vi "test4.2-AsyncMessageWithReply_Queue.vi"(8 "error in (no error)":errorcluster, 11 "TestCase in":refnum<class "testcase-CSMGlobalLog.lvclass">) -> (0 "error out":errorcluster, 3 "TestCase out":refnum<class "testcase-CSMGlobalLog.lvclass">)   [LabVIEW 2017, in "testcase-CSMGlobalLog.lvclass"]
uses:
  testcase-CSMGlobalLog.lvclass
  testcase-CSMGlobalLog.lvclass/testcase-CSMGlobalLog.ctl
  c9cb4a92-c6b2-48ff-9945-b938079fd949.vi
  <vilib>/addons/_JKI Toolkits/VI Tester/TestCase.llb/TestCase.lvclass
  src/user.lib/_NEVSTOP/Communicable State Machine(CSM)/Communicable State Machine.lvlib
  src/user.lib/_NEVSTOP/Communicable State Machine(CSM)/Utility/Periodic String Filter Setting.ctl
  C:/Program Files (x86)/National Instruments/LabVIEW 2017/vi.lib/addons/_JKI Toolkits/VI Tester/TestCase.llb/TestCase.lvclass
panel:
  out "String cache total":string
  out "size(s)":i32
  out "error out 2":errorcluster
  out "LoopCount":i32
  out "String Cache each loop":string
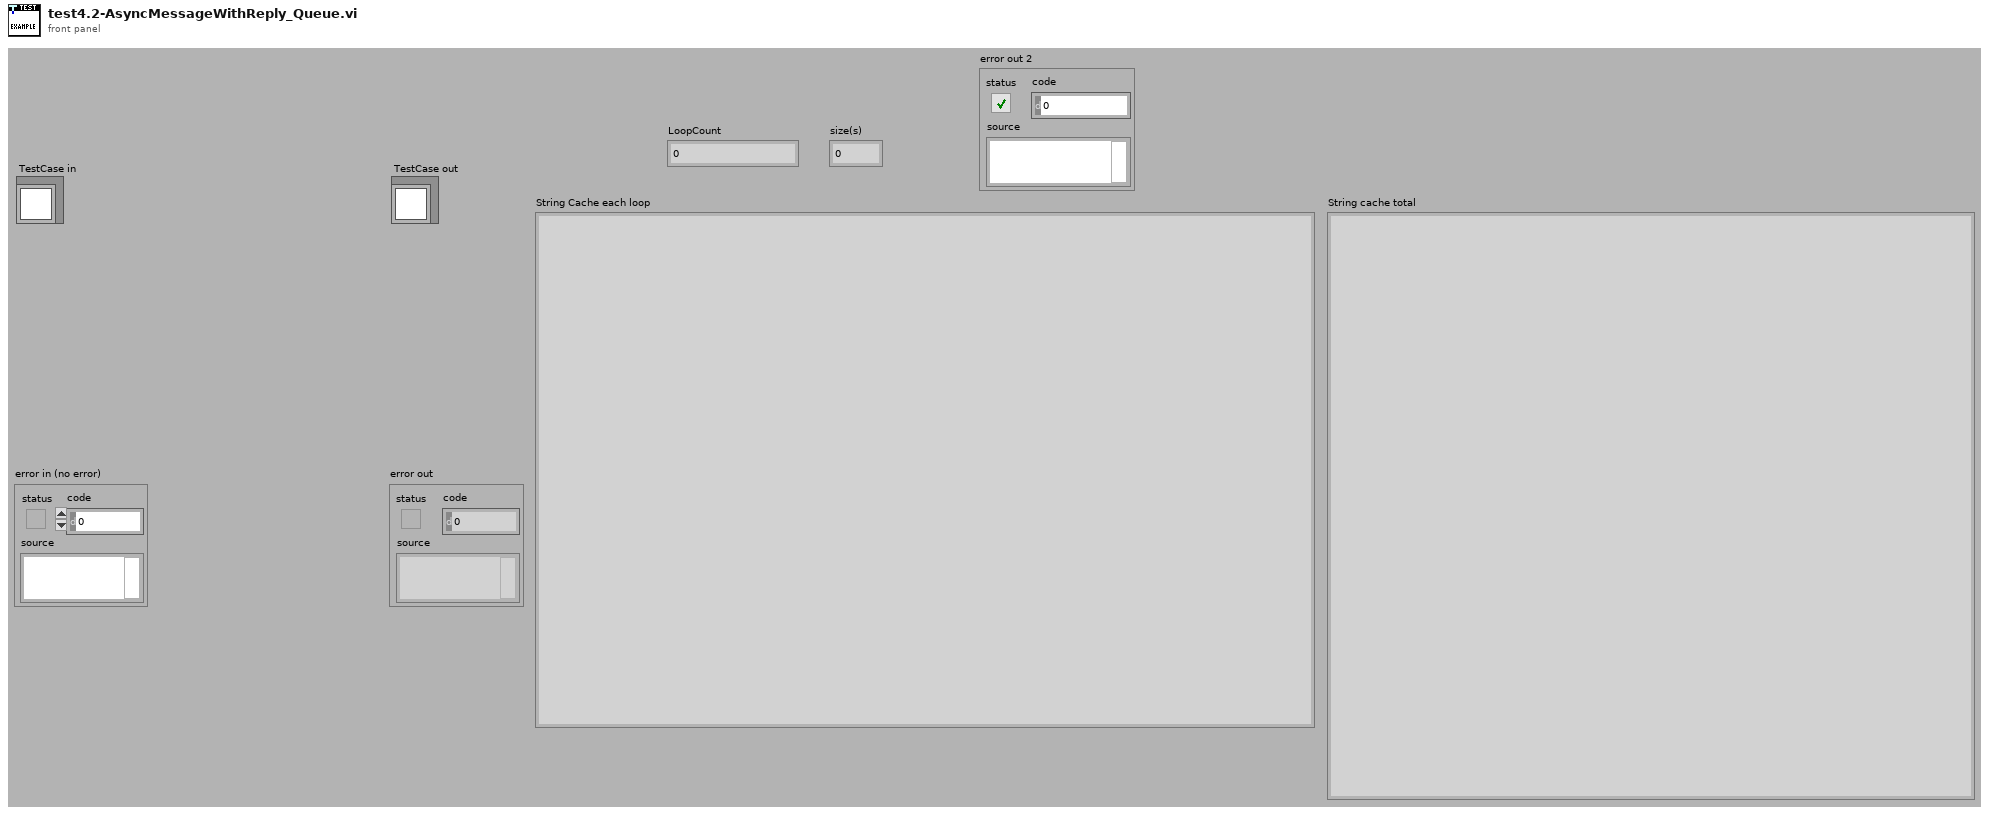
[diagram p1: front panel]
types:
  T1 = typedef "Communicable State Machine.lvlib/Periodic String Filter Setting.ctl" = cluster{"threashold(#/s)":dbl, "Check Peroid(s)":dbl}
  T2 = typedef "Communicable State Machine.lvlib/_CSM_GlobalLog_MSG.ctl" = cluster{"Name (\"\" to Use UUID)":string, "Current State":string, "Arguments":string, "Source Message":T3, "Source Module":string, "Complete(T)/Start(F)":bool, "LogType":T4, "Time Stamp":timestamp}
  T3 = typedef "Communicable State Machine.lvlib/_CSM_Response Source Message.ctl" = cluster{"‘State":string, "’Arguments":string, "’Error":errorcluster}
  T4 = typedef "Communicable State Machine.lvlib/_CSM_GlobalLog_MSG_TYPE.ctl" = enum16{"User Log", "State Change", "Status", "Interrupt", "Register", "Unregister", "Error Log", "Module Created", "Module Destroyed", "Async Message", "No-Rep Async Message", "Sync Message"}
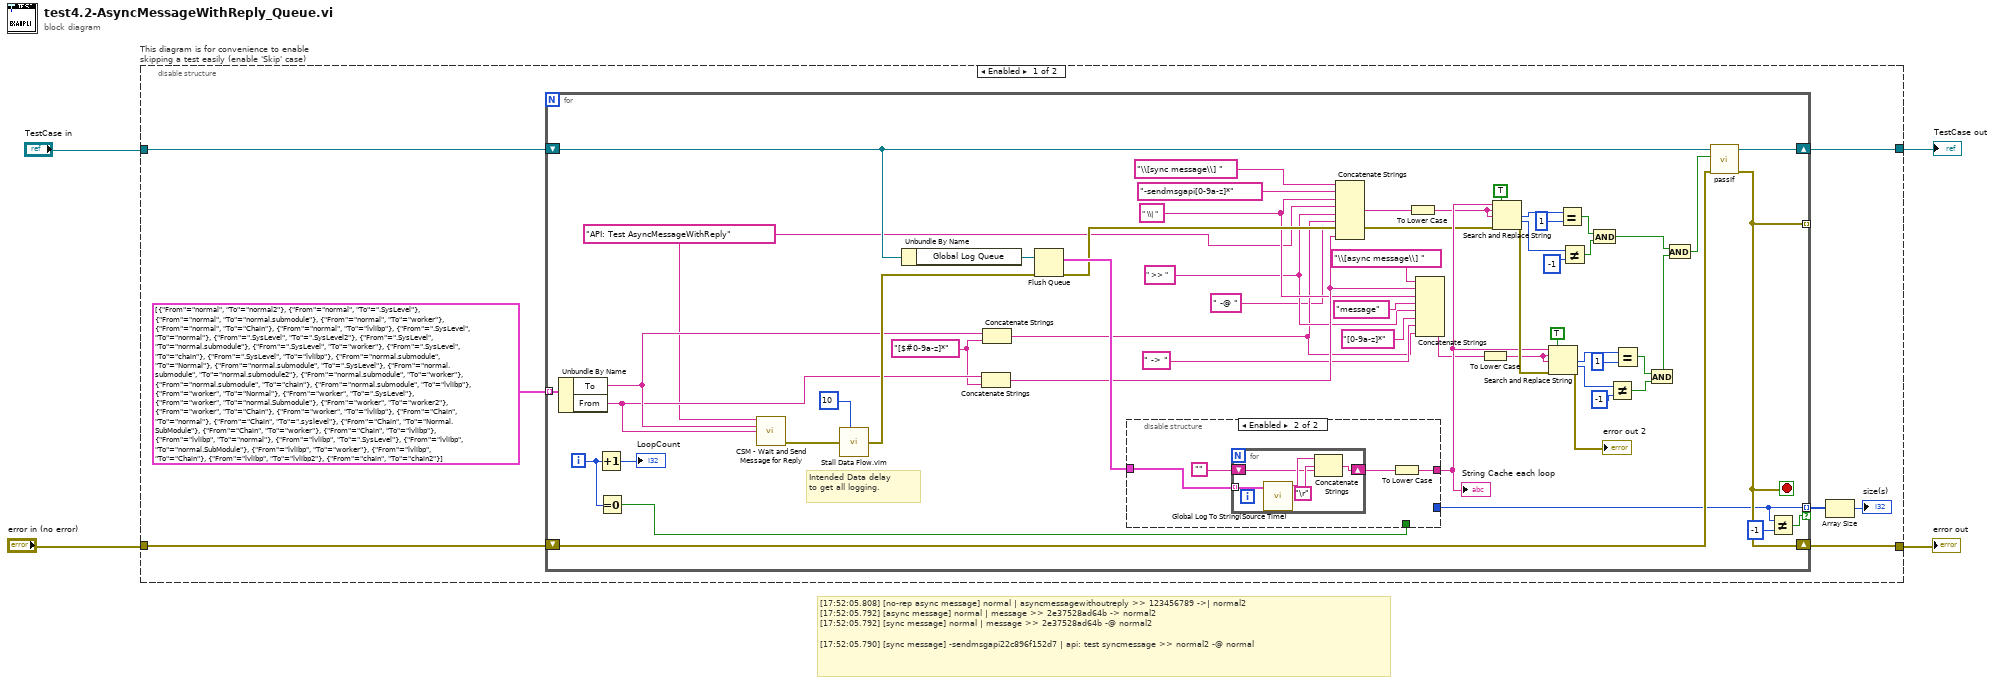
[diagram p0: block diagram]
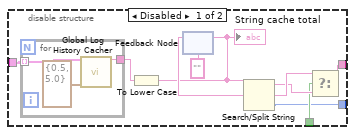
[diagram p2: hidden frame]
diagram:
  # "[17:52:05.808] [no-rep async message] normal | asyncmessagewithoutreply >> 123456789 ->| normal2\n[17:52:05.792] [async message] normal | message >> 2e37528ad64b -> normal2\n[17:52:05.792] [sync message] normal | message >> 2e37528ad64b -@ normal2\n\n[17:52:05.790] [sync message] -sendmsgapi22c896f152d7 | api: test syncmessage >> normal2 -@ normal"
  n1 = disable-structure "This diagram is for convenience to enable skipping a test easily (enable 'Skip' case)" shown="Enabled" {
    disable-tunnel: "TestCase in" -> [w8 w93]
    disable-tunnel: [w10 w91] -> w1
    disable-tunnel: [w11 w92] -> w3
    disable-tunnel: "error in (no error)" -> [w9 w90]
    frame Enabled {
      n2 = for {
        tunnel: cluster{"From":string, "To":string}[] [{"From"="normal", "To"="normal2"}, {"From"="normal", "To"=".SysLevel"}, {"From"="normal", "To"="normal.submodule"}, {"From"="normal", "To"="worker"}, {"From"="normal", "To"="Chain"}, {"From"="normal", "To"="lvlibp"}, {"From"=".SysLevel", "To"="normal"}, {"From"=".SysLevel", "To"=".SysLevel2"}, {"From"=".SysLevel", "To"="normal.submodule"}, {"From"=".SysLevel", "To"="worker"}, {"From"=".SysLevel", "To"="chain"}, {"From"=".SysLevel", "To"="lvlibp"}, {"From"="normal.submodule", "To"="Normal"}, {"From"="normal.submodule", "To"=".SysLevel"}, {"From"="normal.submodule", "To"="normal.submodule2"}, {"From"="normal.submodule", "To"="worker"}, {"From"="normal.submodule", "To"="chain"}, {"From"="normal.submodule", "To"="lvlibp"}, {"From"="worker", "To"="Normal"}, {"From"="worker", "To"=".SysLevel"}, {"From"="worker", "To"="normal.Submodule"}, {"From"="worker", "To"="worker2"}, {"From"="worker", "To"="Chain"}, {"From"="worker", "To"="lvlibp"}, {"From"="Chain", "To"="normal"}, {"From"="Chain", "To"=".syslevel"}, {"From"="Chain", "To"="Normal.SubModule"}, {"From"="Chain", "To"="worker"}, {"From"="Chain", "To"="lvlibp"}, {"From"="lvlibp", "To"="normal"}, {"From"="lvlibp", "To"=".SysLevel"}, {"From"="lvlibp", "To"="normal.SubModule"}, {"From"="lvlibp", "To"="worker"}, {"From"="lvlibp", "To"="Chain"}, {"From"="lvlibp", "To"="lvlibp2"}, {"From"="chain", "To"="chain2"}] -> [w45] mode=indexing
        shift-right: [w43] -> w11
        shift-left: w9 -> [w65]
        shift-right: [w67] -> w10
        shift-left: w8 -> [w44]
        tunnel: [w43] -> _ mode=indexing
        tunnel: [w32] -> w6 mode=indexing if=w42
        i -> [w40]
        stop <- w43 stop-if-true
        w12 = "[$#0-9a-z]*" ("string")
        w23 = " >> "
        w25 = " \\| "
        w15 = "API: Test AsyncMessageWithReply" ("State")
        # "Intended Data delay\nto get all logging."
        n3 = Unbundle By Name(w45) -> ("To"=w29:string, "From"=w28:string)
        n4 = Increment(x=w40) -> (x+1=→"LoopCount":i32)
        n5 = Equal To 0?(x=w40) -> (x = 0?=w33:bool)
        n6 = call "CSM - Wait and Send Message for Reply.vi"("State"=w15, "Arguments (\"\")"=w29, "Target Module"=w28) -> ("error out"=w39:errorcluster)  [unwired: 10 in, 2 out]
        n7 = call "Stall Data Flow.vim"("value in"=w39, "milliseconds to wait"=u32 10 ("millisecond timer value")) -> ("value out"=w38:errorcluster)  [unwired: 1 out]
        n8 = Unbundle By Name(w44) -> ("Global Log Queue"=w66:refnum<queue>)
        n9 = Concatenate Strings(w28, w12) -> (w26:string)
        n10 = Concatenate Strings(w29, w12) -> (w20:string)
        n11 = Flush Queue(queue=w66, error in (no error)=w38) -> (remaining elements=w35:T2[], error out=w31:errorcluster)  [unwired: 1 out]
        n12 = disable-structure shown="Enabled" {
          disable-tunnel: [w71 w81] -> w34
          disable-tunnel: w33 -> [w70 _]
          disable-tunnel: w35 -> [w69 w83]
          disable-tunnel: [w68 _] -> w32
          frame Disabled {
            n13 = for {
              tunnel: w69 -> [w80] mode=indexing
              tunnel: [w79] -> w77
              n14 = call "Global Log History Cacher.vi"("Global Log Data"=w80, "Settings"=T1 {"threashold(#/s)"=0.5, "Check Peroid(s)"=5.0}) -> ("String Cache"=w79:string)  [unwired: 13 in]
            }
            n15 = To Lower Case(string=w77) -> (all lower case string=w72:string)
            "String cache total" <- w72
            n16 = feedback #1("") -> (w76:string)
            n17 = feedback-in #1(w72) -> ()
            n18 = Search/Split String(string=w72, search string/char (-)=w76) -> (substring before match=w73:string, match + rest of string=w74:string, offset of match=w68:i32)  [unwired: 1 in]
            n19 = Select(t=w74, s=w70, f=w73) -> (s? t:f=w71:string)
          }
          frame Enabled {
            n20 = for {
              tunnel: w83 -> [w89] mode=indexing
              shift-right: [w85] -> w82
              shift-left: "" -> [w86]
              n21 = call "Global Log To String(Source Time).vi"("Log"=w89) -> ("Log String"=w88:string)  [unwired: 9 in]
              n22 = Concatenate Strings(w88, "\r", w86) -> (w85:string)
            }
            n23 = To Lower Case(string=w82) -> (all lower case string=w81:string)
          }
        }
        "String Cache each loop" <- w34
        n24 = Concatenate Strings("\\[sync message\\] ", "-sendmsgapi[0-9a-z]*", w25, w15, w23, w20, " -@ " ("string"), w26) -> (w19:string)
        n25 = To Lower Case(string=w19) -> (all lower case string=w18:string)
        n26 = Concatenate Strings("\\[async message\\] " ("string"), w26, w25, "message", w23, "[0-9a-z]*", " -> ", w20) -> (w17:string)
        n27 = To Lower Case(string=w17) -> (all lower case string=w16:string)
        n28 = Search and Replace String(replace all?=TRUE ("replace all? (F)"), input string=w34, search string=w18, replace string=w18, error in=w31) -> (number of replacements=w62:i32, offset past replacement=w61:i32, error out=w51:errorcluster)  [unwired: 3 in, 1 out]
        n29 = Search and Replace String(replace all?=TRUE ("replace all? (F)"), input string=w34, search string=w16, replace string=w16, error in=w51) -> (number of replacements=w53:i32, offset past replacement=w54:i32, error out=→"error out 2":errorcluster)  [unwired: 3 in, 1 out]
        n30 = Equal?(x=w62, y=1) -> (x = y?=w59:bool)
        n31 = Not Equal?(x=w61, y=-1) -> (x != y?=w58:bool)
        n32 = And(x=w59, y=w58) -> (x .and. y?=w46:bool)
        n33 = Not Equal?(x=w54, y=-1) -> (x != y?=w57:bool)
        n34 = Equal?(x=w53, y=1) -> (x = y?=w56:bool)
        n35 = And(x=w56, y=w57) -> (x .and. y?=w50:bool)
        n36 = And(x=w46, y=w50) -> (x .and. y?=w36:bool)
        n37 = call-dynamic "passIf.vi"("error in (no error)"=w65, "pass"=w36, "TestCase in"=w44) -> ("error out"=w43:errorcluster, "TestCase out"=w67:refnum<class "testcase-CSMGlobalLog.lvclass">)  [unwired: 7 in]
        n38 = Not Equal?(x=w32, y=-1) -> (x != y?=w42:bool)
      }
      n39 = Array Size(array=w6) -> (size(s)=→"size(s)":i32)
    }
    frame Disabled {
      # "skip test result while test is under development"
      n40 = call <vilib>:"skip.vi"("error in (no error)"=w90, "TestCase in"=w93) -> ("error out"=w92:errorcluster, "TestCase out"=w91:refnum<class "testcase-CSMGlobalLog.lvclass">)  [unwired: 8 in]
    }
  }
  "error out" <- w3
  "TestCase out" <- w1
